vi "GEOM_GUI_draw_1amp.vi"(4 "zoom factor":dbl=1.0, 5 "draw contour":bool=TRUE, 6 "picture size":T1, 7 "order":u32, 8 "detnum":bool, 9 "corr amps":T3, 10 "amps":T4={"number"=0, "type"=0, "rotated"=0, "fliped"=0, "FPAcoord"={"xstart"=1, "ystart"=1}, "Physical_size"={"columns"=0, "rows"=0}, "predata"={"columns"=0, "rows"=0}, "postdata"={"columns"=0, "rows"=0}, "Req ROIs"=[], "Corr ROI"=[], "Detnumber"=0, "ampID"="", "discard"=0} {"fliped" items=["none", "horizontal", "vertical"]; "type" items=["LL", "LR", "UL", "UR"]}, 11 "picture in":picture) -> (3 "picture out":picture)   [LabVIEW 2016]
uses:
  private/vis/GEOM_Amplifier.ctl
  private/vis/GEOM_AmpType.ctl
  private/vis/GEOM_ROI.ctl
  private/vis/GEOM_Coords.ctl
  <vilib>/Utility/miscctls.llb/LVBoundsTypeDef.ctl
panel:
  in  "offset":dbl=22.0
  in  "origin":cluster{"x":i16, "y":i16}
  in  "rect":T2
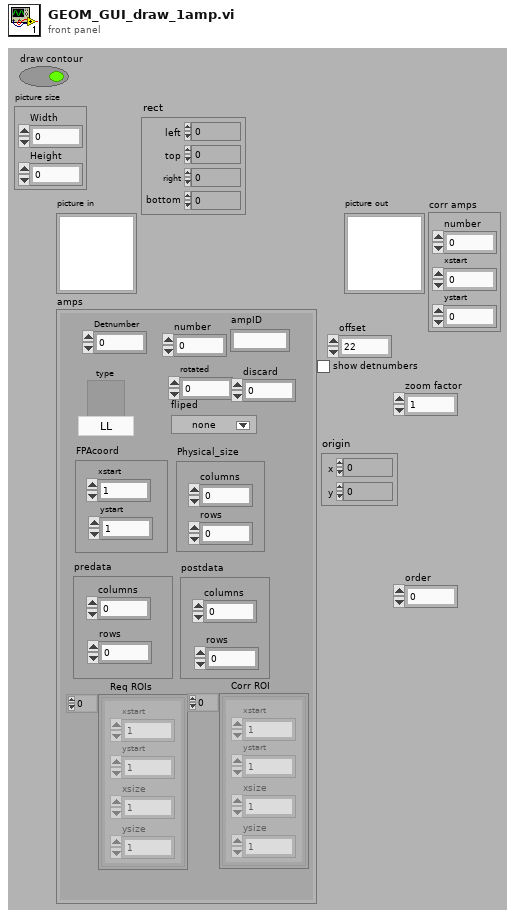
[diagram p1: front panel]
types:
  T1 = typedef "LVBoundsTypeDef.ctl" = cluster{"Width":u32, "Height":u32}
  T2 = cluster{"left":i16, "top":i16, "right":i16, "bottom":i16}
  T3 = cluster{"number":i32, "xstart":i32, "ystart":i32}
  T4 = typedef "GEOM_Amplifier.ctl" = cluster{"number":i32, "type":T5, "rotated":i16, "fliped":u16, "FPAcoord":cluster{"xstart":i32, "ystart":i32}, "Physical_size":cluster{"columns":i32, "rows":i32}, "predata":cluster{"columns":i32, "rows":i32}, "postdata":cluster{"columns":i32, "rows":i32}, "Req ROIs":T6, "Corr ROI":T6, "Detnumber":i32, "ampID":string, "discard":i32}
  T5 = typedef "GEOM_AmpType.ctl" = u16
  T6 = typedef "GEOM_ROI.ctl" = T7[]
  T7 = typedef "GEOM_Coords.ctl" = cluster{"xstart":u32, "ystart":u32, "xsize":u32, "ysize":u32}
  T8 = enum16{"None", "Stacked", "Clockwise", "Counterclockwise"}
  T9 = enum16{"User-specified Font", "Application Font", "System Font", "Dialog Font"}
  T10 = cluster{"Font Name:":string, "Size":i16, "Strikeout?":bool, "Italic?":bool, "Underline?":bool, "Outline?":bool, "Shadow?":bool, "Bold?":bool}
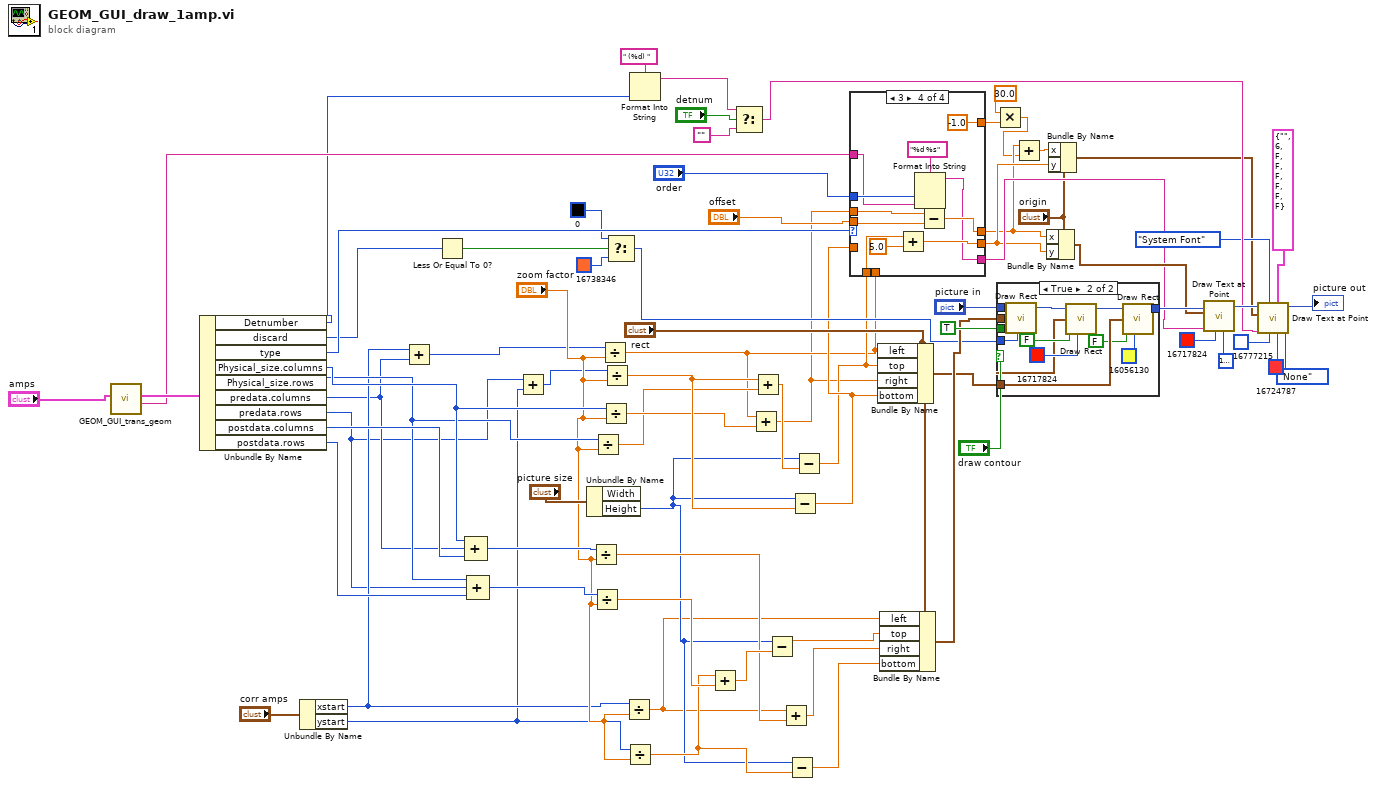
[diagram p0: block diagram]
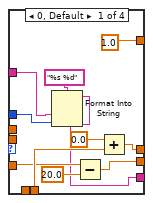
[diagram p3: hidden frame]
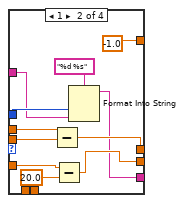
[diagram p4: hidden frame]
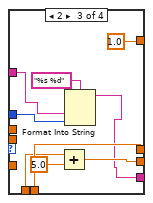
[diagram p5: hidden frame]
diagram:
  n1 = call "GEOM_GUI_trans_geom.vi"("amps in"="amps") -> ("amp direction"=w37:string, "amps out"=w38:T4)  [unwired: 9 out]
  n2 = Unbundle By Name(w38) -> ("Detnumber"=w29:i32, "discard"=w36:i32, "type"=w46:T5, "Physical_size.columns"=w62:i32, "Physical_size.rows"=w61:i32, "predata.columns"=w51:i32, "predata.rows"=w48:i32, "postdata.columns"=w67:i32, "postdata.rows"=w66:i32)
  n3 = Unbundle By Name("corr amps") -> ("xstart"=w52:i32, "ystart"=w49:i32)
  n4 = Add(x=w52, y=w51) -> (x+y=w50:i32)
  n5 = Less Or Equal To 0?(x=w36) -> (x <= 0?=w35:bool)
  n6 = Compound Arithmetic op=ADD(w62, w51, w67) -> (w65:i32)
  n7 = Compound Arithmetic op=ADD(w61, w48, w66) -> (w64:i32)
  n8 = Add(x=w48, y=w49) -> (x+y=w47:i32)
  n9 = Unbundle By Name("picture size") -> ("Height"=w45:u32)  [unwired: 1 out]
  n10 = Divide(x=w65, y="zoom factor") -> (x/y=w57:dbl)
  n11 = Divide(x=w64, y="zoom factor") -> (x/y=w59:dbl)
  n12 = Divide(x=w61, y="zoom factor") -> (x/y=w68:dbl)
  n13 = Divide(x=w50, y="zoom factor") -> (x/y=w12:dbl)
  n14 = Divide(x=w62, y="zoom factor") -> (x/y=w69:dbl)
  n15 = Divide(x=w47, y="zoom factor") -> (x/y=w70:dbl)
  n16 = Select(t=u32 0 ("color(black)"), s=w35, f=u32 16738346 ("color(black)")) -> (s? t:f=w33:u32)
  n17 = Divide(x=w52, y="zoom factor") -> (x/y=w9:dbl)
  n18 = Divide(x=w49, y="zoom factor") -> (x/y=w56:dbl)
  n19 = Format Into String(format string=" (%d) ", w29) -> (resulting string=w28:string)  [unwired: 2 in, 1 out]
  n20 = Add(x=w56, y=w59) -> (x+y=w58:dbl)
  n21 = Select(t=w28, s="detnum", f="") -> (s? t:f=w21:string)
  n22 = Add(x=w12, y=w69) -> (x+y=w11:dbl)
  n23 = Add(x=w70, y=w68) -> (x+y=w72:dbl)
  n24 = Subtract(x=w45, y=w58) -> (x-y=w15:dbl)
  n25 = Add(x=w9, y=w57) -> (x+y=w10:dbl)
  n26 = Subtract(x=w45, y=w56) -> (x-y=w16:dbl)
  n27 = Subtract(x=w45, y=w70) -> (x-y=w14:dbl)
  n28 = Subtract(x=w45, y=w72) -> (x-y=w13:dbl)
  n29 = case shown="3" w46 {
    tunnel: [w77 w91 w99 w111] -> w26
    tunnel: [w85 w94 w106 w115] -> w5
    tunnel: [w83 w96 w104 w114] -> w7
    tunnel: w13 -> [_ _ w105 w117]
    tunnel: w12 -> [w86 _ w106 _]
    tunnel: w11 -> [_ w95 _ w116]
    tunnel: w14 -> [w82 w97 _ _]
    tunnel: "order" -> [w79 w93 w101 w113]
    tunnel: "offset" -> [_ w90 _ w110]
    tunnel: w37 -> [w78 w88 w100 w108]
    tunnel: [1.0 ("y") -1.0 ("y") 1.0 ("y") -1.0 ("y")] -> w2
    frame 0, Default {
      n30 = Format Into String(format string="%s %d", w78, w79) -> (resulting string=w77:string)  [unwired: 2 in, 1 out]
      n31 = Subtract(x=w82, y=20.0) -> (x-y=w83:dbl)
      n32 = Add(x=0.0, y=w86) -> (x+y=w85:dbl)
    }
    frame 1 {
      n33 = Subtract(x=w95, y=w90) -> (x-y=w94:dbl)
      n34 = Subtract(x=w97, y=20.0) -> (x-y=w96:dbl)
      n35 = Format Into String(format string="%d %s", w93, w88) -> (resulting string=w91:string)  [unwired: 2 in, 1 out]
    }
    frame 2 {
      n36 = Add(x=w105, y=5.0) -> (x+y=w104:dbl)
      n37 = Format Into String(format string="%s %d", w100, w101) -> (resulting string=w99:string)  [unwired: 2 in, 1 out]
    }
    frame 3 {
      n38 = Add(x=w117, y=5.0) -> (x+y=w114:dbl)
      n39 = Format Into String(format string="%d %s", w113, w108) -> (resulting string=w111:string)  [unwired: 2 in, 1 out]
      n40 = Subtract(x=w116, y=w110) -> (x-y=w115:dbl)
    }
  }
  n41 = Bundle By Name(cluster="rect", "left"=w12, "top"=w13, "right"=w11, "bottom"=w14) -> (w54:T2)
  n42 = Bundle By Name(cluster="rect", "left"=w9, "top"=w15, "right"=w10, "bottom"=w16) -> (w55:T2)
  n43 = Multiply(x=30.0 ("y"), y=w2) -> (x*y=w3:dbl)
  n44 = case shown="True" "draw contour" {
    tunnel: "picture in" -> [w118 w130]
    tunnel: TRUE ("fill?(F)") -> [_ w129]
    tunnel: w55 -> [_ w125]
    tunnel: w54 -> [_ w123]
    tunnel: [w118 w120] -> w53
    tunnel: w33 -> [_ w119]
    frame False {
    }
    frame True {
      n45 = call <vilib>:"Draw Rect.vi"("picture"=w130, "rect"=w125, "fill?(F)"=w129, "color(black)"=w119) -> ("new picture"=w128:picture)  [unwired: 1 in, 4 out]
      n46 = call <vilib>:"Draw Rect.vi"("picture"=w128, "rect"=w125, "fill?(F)"=FALSE, "color(black)"=u32 16717824) -> ("new picture"=w124:picture)  [unwired: 1 in, 4 out]
      n47 = call <vilib>:"Draw Rect.vi"("picture"=w124, "rect"=w123, "fill?(F)"=FALSE, "color(black)"=u32 16056130) -> ("new picture"=w120:picture)  [unwired: 1 in, 4 out]
    }
  }
  n48 = Add(x=w5, y=w3) -> (x+y=w6:dbl)
  n49 = Bundle By Name(cluster="origin", "x"=w5, "y"=w7) -> (w42:cluster{"x":i16, "y":i16})
  n50 = Bundle By Name(cluster="origin", "x"=w6, "y"=w7) -> (w17:cluster{"x":i16, "y":i16})
  n51 = call <vilib>:"Draw Text at Point.vi"("BG color(transparent)"=u32 16777216, "text color(black)"=u32 16717824, "text"=w26, "origin"=w42, "picture"=w53) -> ("new picture"=w25:picture)  [unwired: 4 in, 2 out]
  n52 = call <vilib>:"Draw Text at Point.vi"("text orientation"=T8."None", "BG color(transparent)"=u32 16724787, "[user-specified font]"=T10 {"Font Name:"="", "Size"=6, "Strikeout?"=FALSE, "Italic?"=FALSE, "Underline?"=FALSE, "Outline?"=FALSE, "Shadow?"=FALSE, "Bold?"=FALSE}, "text color(black)"=u32 16777215, "desired font(Application)"=T9."System Font", "text"=w21, "origin"=w17, "picture"=w25) -> ("new picture"=→"picture out":picture)  [unwired: 1 in, 2 out]
